vi "PID.vi"(0 "heat_board_control in":refnum<class "heat_board_control.lvclass">, 5 "Waveform":waveform(dbl), 7 "millisecond multiple":u32, 9 "Lock All":bool, 11 "error in (no error)":errorcluster) -> (4 "heat_board_control out":refnum<class "heat_board_control.lvclass">, 6 "data average":dbl, 8 "PD setpoint":dbl, 10 "laser setpoint":dbl, 15 "error out":errorcluster)   [LabVIEW 2015, in "heat_board_control.lvclass"]
uses:
  heat_board_control.lvclass
  <vilib>/Analysis/baseanly.llb/Mean (DBL).vi
  <vilib>/addons/control/pid/pid.llb/PID (DBL).vi
  <vilib>/addons/control/pid/NI_PID_pid.lvlib
  <vilib>/Analysis/NI_AALBase.lvlib
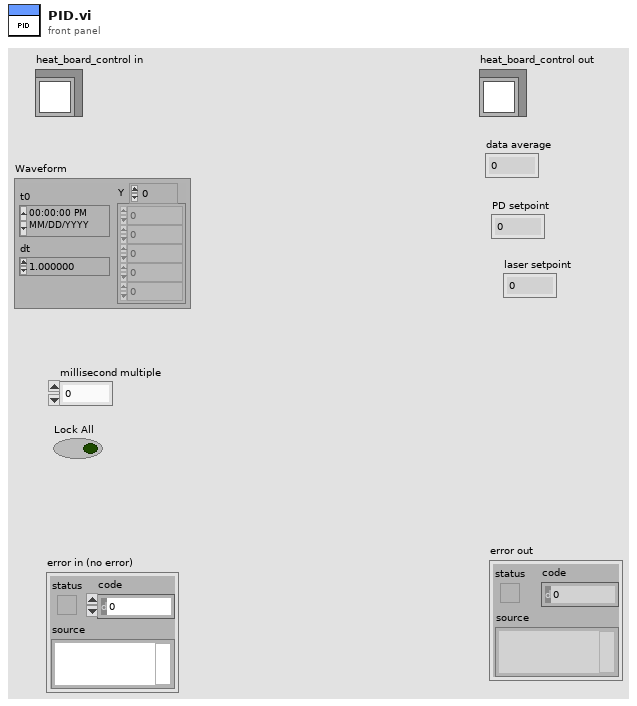
[diagram p1: front panel]
types:
  T1 = cluster{"proportional gain (Kc)":dbl, "derivative time (Td, min)":dbl, "integral time (Ti, min)":dbl}
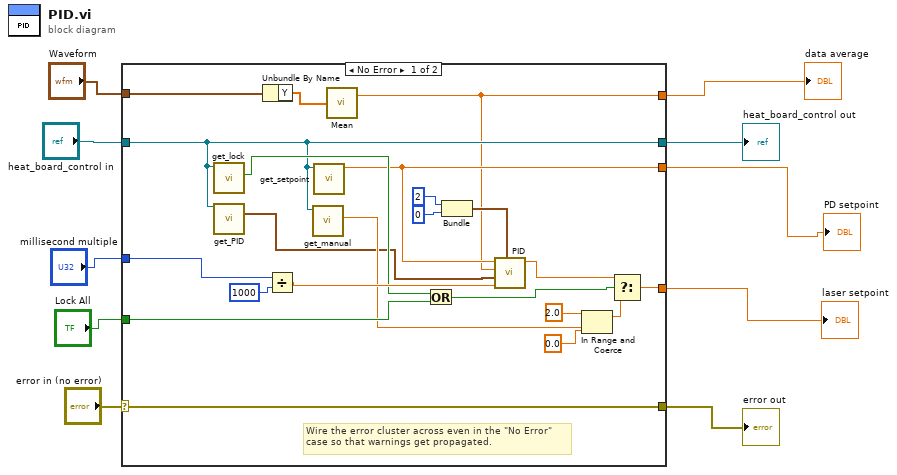
[diagram p0: block diagram]
diagram:
  n1 = case shown="No Error" "error in (no error)" {
    selector: "error in (no error)" -> [w32 w34]
    tunnel: [w32 w34] -> w9
    tunnel: [w21 w33] -> w7
    tunnel: "heat_board_control in" -> [w21 w33]
    tunnel: "Waveform" -> [w27 _]
    tunnel: "millisecond multiple" -> [w26 _]
    tunnel: "Lock All" -> [w25 _]
    tunnel: [w12 _] -> w3
    tunnel: [w23 _] -> w2
    tunnel: [w11 _] -> w1
    frame No Error {
      # "Wire the error cluster across even in the \"No Error\"\ncase so that warnings get propagated."
      n2 = call-dynamic "get_lock.vi"("heat_board_control in"=w21) -> ("Boolean"=w24:bool)  [unwired: 8 in, 2 out]
      n3 = call-dynamic "get_PID.vi"("heat_board_control in"=w21) -> ("Cluster"=w20:T1)  [unwired: 12 in, 2 out]
      n4 = Unbundle By Name(w27) -> ("Y"=w13:dbl[])
      n5 = Divide(x=w26, y=u32 1000) -> (x/y=w29:dbl)
      n6 = call-dynamic "get_manual.vi"("heat_board_control in"=w21) -> ("setpoint"=w22:dbl)  [unwired: 8 in, 2 out]
      n7 = call-dynamic "get_setpoint.vi"("heat_board_control in"=w21) -> ("setpoint"=w23:dbl)  [unwired: 8 in, 2 out]
      n8 = call-poly <vilib>:"Mean.vi"("X"=w13) -> ("mean"=w12:dbl)  [unwired: 1 out]
      n9 = Or(x=w24, y=w25) -> (x .or. y?=w30:bool)
      n10 = Bundle(2, 0) -> (w16:cluster{i32, i32})  [unwired: 1 in]
      n11 = call-poly <vilib>:"PID.vi"("output range"=w16, "dt (s)"=w29, "PID gains"=w20, "process variable"=w12, "setpoint"=w23) -> ("output"=w31:dbl)  [unwired: 5 in, 1 out]
      n12 = In Range and Coerce(upper limit=2.0, x=w22, lower limit=0.0) -> (coerced(x)=w19:dbl)  [unwired: 1 out]
      n13 = Select(t=w31, s=w30, f=w19) -> (s? t:f=w11:dbl)
    }
    frame Error {
    }
  }
  "error out" <- w9
  "heat_board_control out" <- w7
  "data average" <- w3
  "PD setpoint" <- w2
  "laser setpoint" <- w1
